vi "_GetEvent.vi"(8 "error in (no error)":errorcluster, 10 "Index":i32, 11 "EventBag in":refnum<class "EventBag.lvclass">) -> (0 "error out":errorcluster, 1 "Item found?":bool, 2 "Event":refnum<class "Event.lvclass">, 3 "EventBag out":refnum<class "EventBag.lvclass">)   [LabVIEW 2021, in "EventManagerLibrary.lvlib" / "EventBag.lvclass"]
uses:
  EventBag.lvclass
  EventObject/Event.lvclass
  EventBag.lvclass/EventBag.ctl
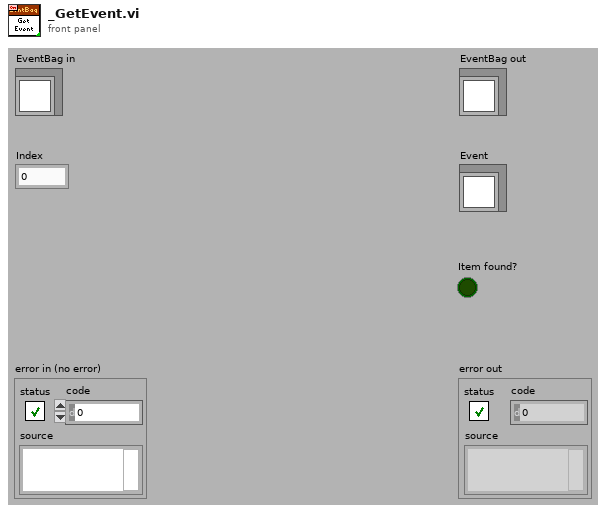
[diagram p1: front panel]
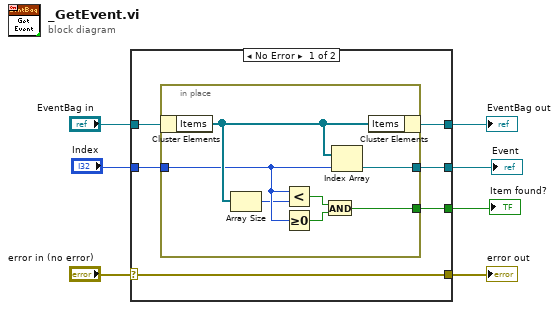
[diagram p0: block diagram]
diagram:
  n1 = case shown="No Error" "error in (no error)" {
    selector: "error in (no error)" -> [w13 w22]
    tunnel: [w13 w22] -> w6
    tunnel: [w11 w21] -> w4
    tunnel: "EventBag in" -> [w12 w21]
    tunnel: "Index" -> [w10 _]
    tunnel: [w9 _] -> w2
    tunnel: [w8 _] -> w1
    frame No Error {
      n2 = in-place {
        in-place-border: w10 -> [w18]
        in-place-border: [w20] -> w9
        in-place-border: [w14] -> w8
        n3 = in-place-cluster #1(w12) -> ("Items"=w19:refnum<class "Event.lvclass">[])
        n4 = Array Size(array=w19) -> (size(s)=w17:i32)
        n5 = Less?(x=w18, y=w17) -> (x < y?=w16:bool)
        n6 = Greater Or Equal To 0?(x=w18) -> (x >= 0?=w15:bool)
        n7 = And(x=w16, y=w15) -> (x .and. y?=w14:bool)
        n8 = Index Array(array=w19, index=w18) -> (element=w20:refnum<class "Event.lvclass">)
        n9 = in-place-cluster #1("Items"=w19) -> (w11:refnum<class "EventBag.lvclass">)
      }
    }
    frame Error {
    }
  }
  "error out" <- w6
  "EventBag out" <- w4
  "Event" <- w2
  "Item found?" <- w1
